vi "Re-PopulateConfigKeyEnum.vi"(8 "error in":errorcluster, 11 "ini file path in":path=path "C:/Documents and Settings/All Users/Application Data/NRS_RX_and_DC_Control/NRS_RX_and_DC_Control.ini") -> (0 "error out":errorcluster, 2 "Sections/Keys/Values":T2(array[cluster]), 3 "ini file path out":path)   [LabVIEW 2013]
doc: "Run this VI after adding new Sections and/or Keys to your configuration file. This will refresh the associated Type Def, so that the new Keys will be available from Type Def constants DURING DEVELOPMENT."
panel:
  out "Keys":T1(ring)
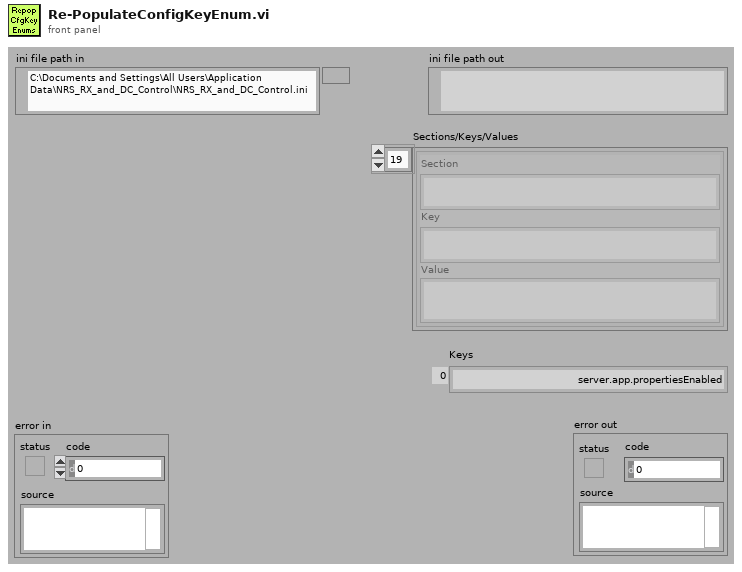
[diagram p1: front panel]
types:
  T1 = enum16{"server.app.propertiesEnabled", "server.ole.enabled", "server.tcp.servic", "server.vi.propertiesEnabled", "WebServer.DirectoryIndex", "WebServer.LogPath", "WebServer.MimeTypes", "WebServer.RootPath", "WebServer.TcpAccess", "WebServer.ViAccess", "NRS.OutputDataFolderPath", "NRS.SwVersionsFilePath", "NRS.Default.PRN", "Default.ReceiverMask", "SymbCap.OutputDataFolderPath", "Default.IpAddress", "Default.StartingTcpPort"}
  T2 = cluster{"Section":string, "Key":string, "Value":string}[]
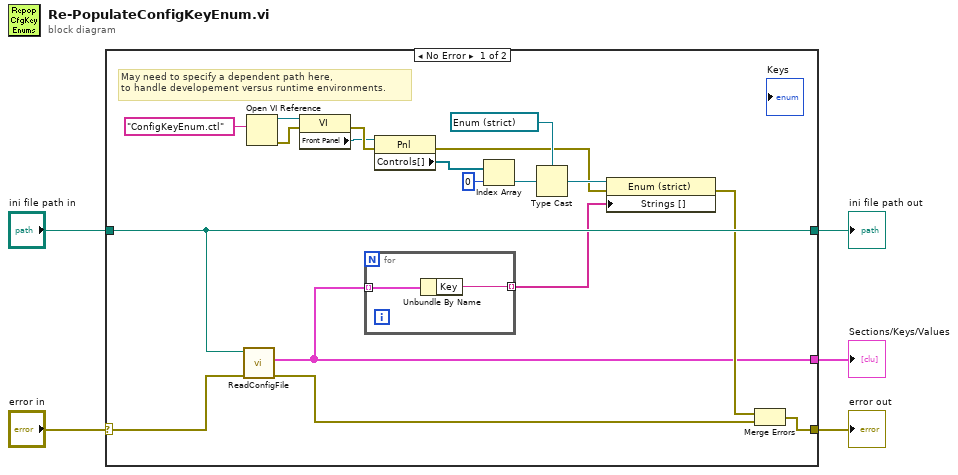
[diagram p0: block diagram]
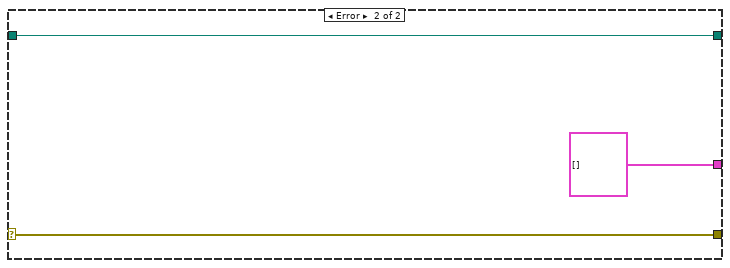
[diagram p2: hidden frame]
diagram:
  n1 = case shown="No Error" "error in" {
    selector: "error in" -> [w22 w28]
    tunnel: "ini file path in" -> [w23 w26]
    tunnel: [w9 T2 []] -> w4
    tunnel: [w11 w28] -> w2
    tunnel: [w23 w26] -> w1
    frame No Error {
      # "May need to specify a dependent path here, \nto handle developement versus runtime environments."
      n2 = call "ReadConfigFile.vi"("error in"=w22, "ini file path in"=w23) -> ("error out"=w10:errorcluster, "Sections/Keys/Values"=w9:T2)  [unwired: 7 in, 1 out]
      n3 = Open VI Reference(vi path="ConfigKeyEnum.ctl") -> (vi reference=w18:refnum<vi>, error out=w20:errorcluster)  [unwired: 5 in]
      n4 = property class="VI"(reference=w18, error in=w20) -> (error out=w21:errorcluster, "Front Panel"=w17:refnum<vi>)  [unwired: 1 out]
      n5 = for {
        tunnel: w9 -> [w25] mode=indexing
        tunnel: [w24] -> w8 mode=indexing
        n6 = Unbundle By Name(w25) -> ("Key"=w24:string)
      }
      n7 = property class="Pnl"(reference=w17, error in=w21) -> (error out=w6:errorcluster, "Controls[]"=w16:refnum<vi>[])  [unwired: 1 out]
      n8 = Index Array(array=w16, index=0) -> (element=w13:refnum<vi>)
      n9 = Type Cast(type=refnum<vi> refnum ("Ctrl Reference"), x=w13) -> (*(type *) &x=w14:refnum<vi>)
      n10 = property class="Enum (strict)"(reference=w14, error in=w6, "Strings []"=w8) -> (error out=w15:errorcluster)  [unwired: 1 out]
      n11 = Merge Errors(w15, w10) -> (w11:errorcluster)
    }
    frame Error {
    }
  }
  "Sections/Keys/Values" <- w4
  "error out" <- w2
  "ini file path out" <- w1
